vi "Get Plots Scale Indices.vi"(8 "Error In":errorcluster, 9 "Y Scale Labels":string[](array[string]), 10 "X Scale Labels":string[](array[string]), 11 "Plot Scales Array":T1[](array[typedef])) -> (0 "Error Out":errorcluster, 3 "Array of Scales (Default)":cluster{"X Scale":u32, "Y Scale":u32}[](array[cluster]))   [LabVIEW 2021, in "Graphs.lvlib"]
uses:
  XY Graph/XY Graph Plot Scale Labels.ctl
  Graphs.lvlib
  XY Graph/XY Graph Add-Ons.lvlib
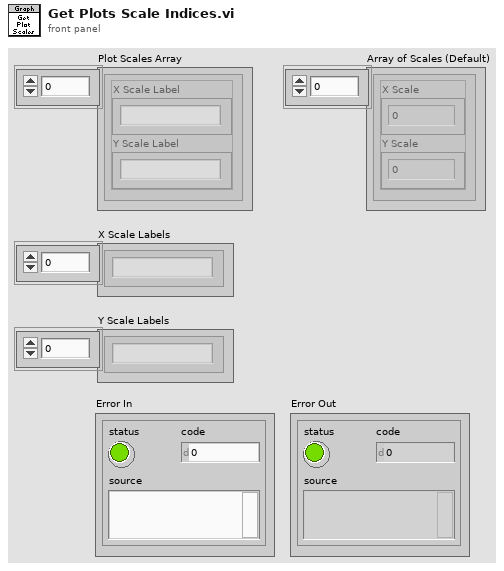
[diagram p1: front panel]
types:
  T1 = typedef "XY Graph Add-Ons.lvlib/XY Graph Plot Scale Labels.ctl" = cluster{"X Scale Label":string, "Y Scale Label":string}
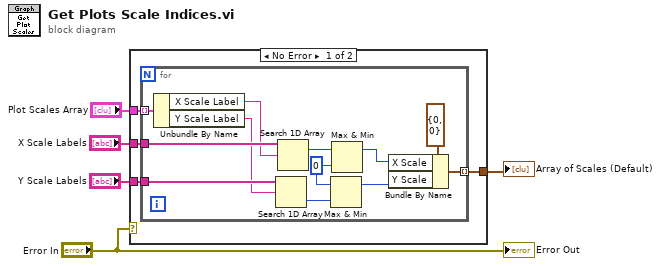
[diagram p0: block diagram]
diagram:
  n1 = case shown="No Error" "Error In" {
    tunnel: "Plot Scales Array" -> [w9 _]
    tunnel: "X Scale Labels" -> [w8 _]
    tunnel: "Y Scale Labels" -> [w7 _]
    tunnel: [w6 _] -> w2
    frame No Error {
      n2 = for {
        tunnel: w9 -> [w21] mode=indexing
        tunnel: w8 -> [w20]
        tunnel: w7 -> [w18]
        tunnel: [w15] -> w6 mode=indexing
        w12 = 0 ("y")
        n3 = Unbundle By Name(w21) -> ("X Scale Label"=w19:string, "Y Scale Label"=w17:string)
        n4 = Search 1D Array(1D array=w18, element=w17) -> (index of element=w13:i32)  [unwired: 1 in]
        n5 = Search 1D Array(1D array=w20, element=w19) -> (index of element=w14:i32)  [unwired: 1 in]
        n6 = Max & Min(x=w12, y=w13) -> (max(x,y)=w10:i32)  [unwired: 1 out]
        n7 = Max & Min(x=w14, y=w12) -> (max(x,y)=w11:i32)  [unwired: 1 out]
        n8 = Bundle By Name(cluster=cluster{"X Scale":u32, "Y Scale":u32} {"X Scale"=0, "Y Scale"=0} ("Cluster"), "X Scale"=w11, "Y Scale"=w10) -> (w15:cluster{"X Scale":u32, "Y Scale":u32})
      }
    }
    frame Error {
    }
  }
  "Array of Scales (Default)" <- w2
  "Error Out" <- "Error In"
